vi "VISA.Open + ID Query.vi"(8 "Error In":errorcluster, 10 "Reset":bool=TRUE, 11 "VISA Name":refnum<visa-resource-name>="FunctGen1") -> (0 "Error Out":errorcluster, 1 "SN":string, 2 "Model":string, 3 "VISA Name Out":refnum<visa-resource-name>, 4 "Rev":string, 5 "Mfg":string)   [LabVIEW 2018]
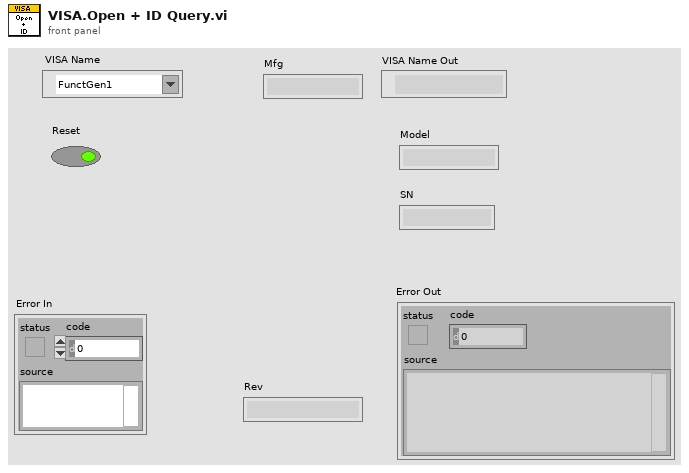
[diagram p1: front panel]
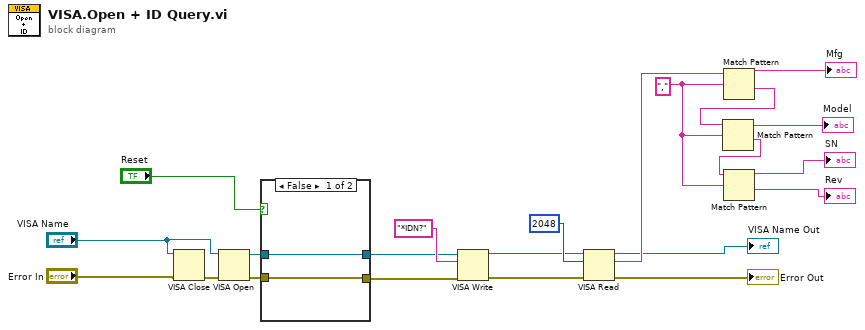
[diagram p0: block diagram]
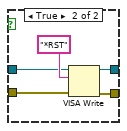
[diagram p2: hidden frame]
diagram:
  w6 = ","
  n1 = VISA Close(VISA resource name="VISA Name", error in (no error)="Error In") -> (error out=w17:errorcluster)
  n2 = VISA Open(error in (no error)=w17, VISA resource name="VISA Name") -> (VISA resource name=w5:refnum<visa-resource-name>, error out=w3:errorcluster)  [unwired: 3 in]
  n3 = case shown="False" "Reset" {
    tunnel: w5 -> [w24 w28]
    tunnel: [w24 w27] -> w4
    tunnel: w3 -> [w23 w26]
    tunnel: [w23 w25] -> w2
    frame False {
    }
    frame True {
      n4 = VISA Write(VISA resource name=w28, write buffer="*RST", error in (no error)=w26) -> (VISA resource name out=w27:refnum<visa-resource-name>, error out=w25:errorcluster)  [unwired: 1 out]
    }
  }
  n5 = VISA Write(VISA resource name=w4, write buffer="*IDN?", error in (no error)=w2) -> (VISA resource name out=w20:refnum<visa-resource-name>, error out=w16:errorcluster)  [unwired: 1 out]
  n6 = VISA Read(VISA resource name=w20, byte count=u32 2048, error in (no error)=w16) -> (VISA resource name out=→"VISA Name Out":refnum<visa-resource-name>, read buffer=w15:string, error out=→"Error Out":errorcluster)  [unwired: 1 out]
  n7 = Match Pattern(string=w15, regular expression=w6) -> (before substring=→"Mfg":string, after substring=w14:string)  [unwired: 1 in, 2 out]
  n8 = Match Pattern(string=w14, regular expression=w6) -> (before substring=→"Model":string, after substring=w9:string)  [unwired: 1 in, 2 out]
  n9 = Match Pattern(string=w9, regular expression=w6) -> (before substring=→"SN":string, after substring=→"Rev":string)  [unwired: 1 in, 2 out]
